vi "error6662.vi"(4 "input error":errorcluster) -> (0 "result":bool, 1 "output error":errorcluster)   [LabVIEW 2010]
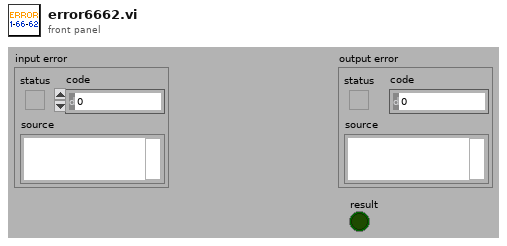
[diagram p1: front panel]
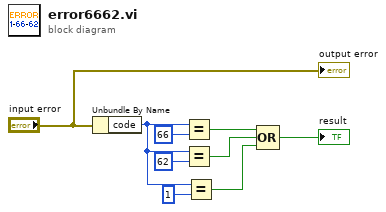
[diagram p0: block diagram]
diagram:
  n1 = Unbundle By Name("input error") -> ("code"=w3:i32)
  n2 = Equal?(x=w3, y=66) -> (x = y?=w6:bool)
  n3 = Equal?(x=w3, y=62) -> (x = y?=w7:bool)
  n4 = Equal?(x=w3, y=1) -> (x = y?=w1:bool)
  n5 = Compound Arithmetic op=OR(w6, w7, w1) -> (→"result":bool)
  "output error" <- "input error"
